vi "Read TSP Net Remote Instrument Data.vi"(7 "Enable Data Check (T: Enable)":bool=TRUE, 8 "error in (no error)":errorcluster, 9 "Data Format (Nil)":string="Nil", 10 "Instrument ID":string, 11 "VISA resource name":refnum<visa-resource-name>) -> (0 "error out":errorcluster, 2 "Remote Data":string, 3 "VISA resource name out":refnum<visa-resource-name>)   [LabVIEW 2017, in "Keithley 2600 Series.lvlib"]
doc: "Returns the data from the remote instrument.\n\n<b>Note:</b>\nThis VI only applies to the TSP-enabled instrument."
uses:
  <instrlib>/Keithley 2600 Series/Keithley 2600 Series.lvlib
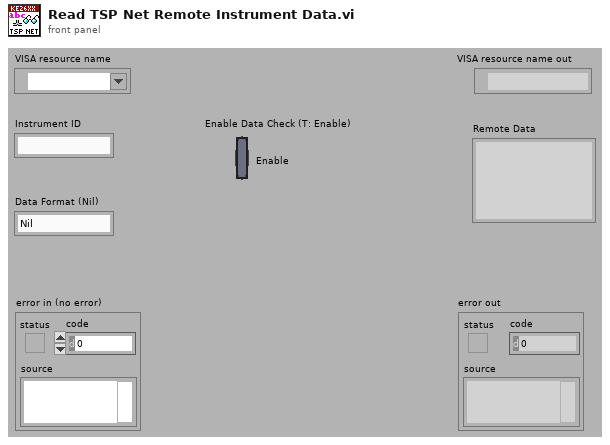
[diagram p1: front panel]
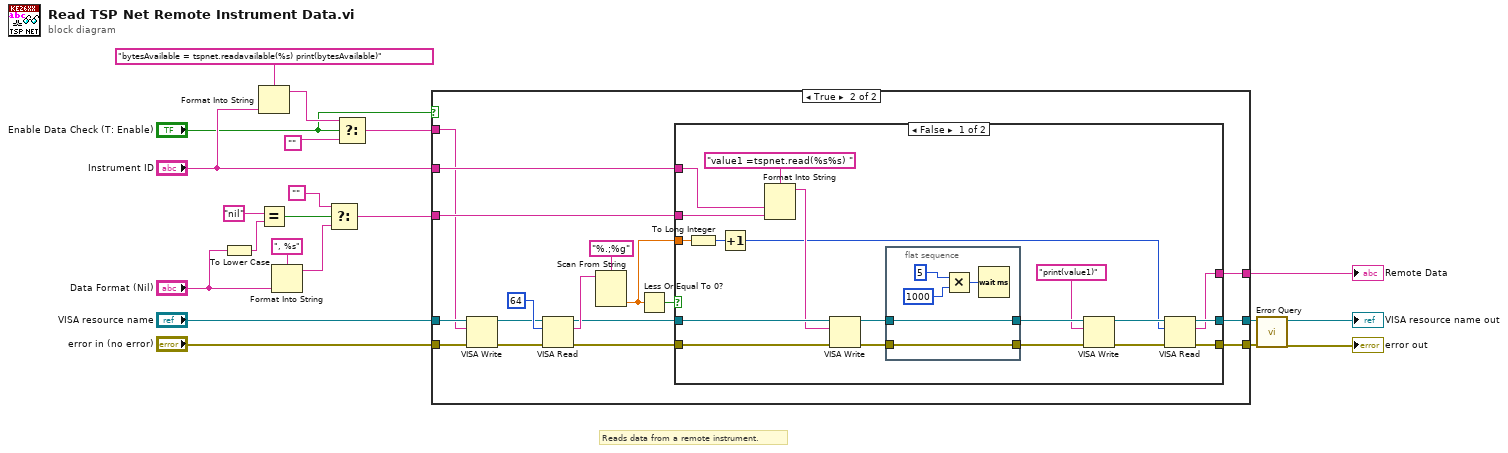
[diagram p0: block diagram]
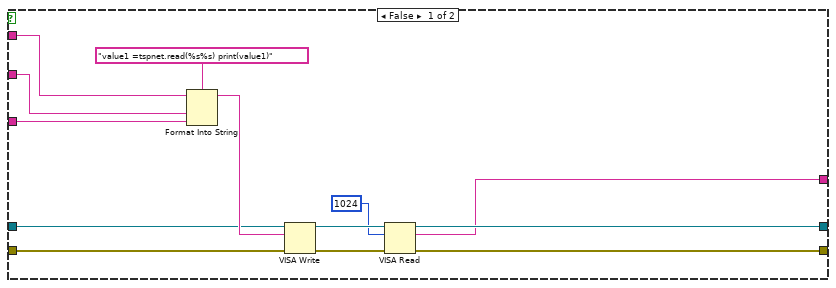
[diagram p2: hidden frame]
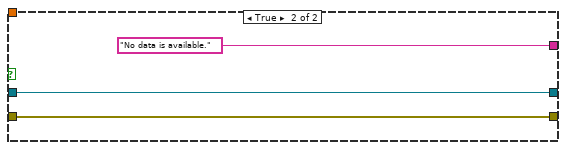
[diagram p3: hidden frame]
diagram:
  # "Reads data from a remote instrument."
  n1 = To Lower Case(string="Data Format (Nil)") -> (all lower case string=w2:string)
  n2 = Format Into String(format string="bytesAvailable = tspnet.readavailable(%s) print(bytesAvailable)", "Instrument ID") -> (resulting string=w18:string)  [unwired: 2 in, 1 out]
  n3 = Equal?(x="nil", y=w2) -> (x = y?=w14:bool)
  n4 = Format Into String(format string=", %s", "Data Format (Nil)") -> (resulting string=w11:string)  [unwired: 2 in, 1 out]
  n5 = Select(t="", s=w14, f=w11) -> (s? t:f=w10:string)
  n6 = Select(t=w18, s="Enable Data Check (T: Enable)", f="") -> (s? t:f=w5:string)
  n7 = case shown="True" "Enable Data Check (T: Enable)" {
    tunnel: "Instrument ID" -> [w23 w45]
    tunnel: w10 -> [w22 w44]
    tunnel: [w27 w43] -> w9
    tunnel: [w26 w42] -> w8
    tunnel: [w25 w41] -> w7
    tunnel: w5 -> [w24 w36]
    tunnel: "VISA resource name" -> [w29 w40]
    tunnel: "error in (no error)" -> [w28 w38]
    frame False {
      n8 = Format Into String(format string="value1 =tspnet.read(%s%s) print(value1)", initial string=w24, w23, w22) -> (resulting string=w30:string)  [unwired: 1 in, 1 out]
      n9 = VISA Write(VISA resource name=w29, write buffer=w30, error in (no error)=w28) -> (VISA resource name out=w33:refnum<visa-resource-name>, error out=w32:errorcluster)  [unwired: 1 out]
      n10 = VISA Read(VISA resource name=w33, byte count=u32 1024, error in (no error)=w32) -> (VISA resource name out=w27:refnum<visa-resource-name>, read buffer=w25:string, error out=w26:errorcluster)  [unwired: 1 out]
    }
    frame True {
      n11 = VISA Write(VISA resource name=w40, write buffer=w36, error in (no error)=w38) -> (VISA resource name out=w39:refnum<visa-resource-name>, error out=w37:errorcluster)  [unwired: 1 out]
      n12 = VISA Read(VISA resource name=w39, byte count=u32 64, error in (no error)=w37) -> (VISA resource name out=w47:refnum<visa-resource-name>, read buffer=w50:string, error out=w46:errorcluster)  [unwired: 1 out]
      n13 = Scan From String(format string="%.;%g", input string=w50) -> (output 1=w35:dbl)  [unwired: 3 in, 3 out]
      n14 = Less Or Equal To 0?(x=w35) -> (x <= 0?=w48:bool)
      n15 = case shown="False" w48 {
        tunnel: w47 -> [w67 w78]
        tunnel: w46 -> [w66 w77]
        tunnel: w45 -> [w69 _]
        tunnel: w44 -> [w68 _]
        tunnel: [w65 w78] -> w43
        tunnel: [w64 w77] -> w42
        tunnel: [w62 "No data is available." ("read buffer")] -> w41
        tunnel: w35 -> [w54 _]
        frame False {
          n16 = To Long Integer(number=w54) -> (32bit integer=w53:i32)
          n17 = Increment(x=w53) -> (x+1=w52:i32)
          n18 = Format Into String(format string="value1 =tspnet.read(%s%s) ", w69, w68) -> (resulting string=w63:string)  [unwired: 2 in, 1 out]
          n19 = VISA Write(VISA resource name=w67, write buffer=w63, error in (no error)=w66) -> (VISA resource name out=w61:refnum<visa-resource-name>, error out=w60:errorcluster)  [unwired: 1 out]
          n20 = flat-sequence {
            tunnel: w61 -> [w75]
            tunnel: w60 -> [w74]
            tunnel: [w75] -> w59
            tunnel: [w74] -> w57
            frame #0 {
              n21 = Multiply(x=5, y=1000) -> (x*y=w73:i32)
              n22 = Wait (ms)(milliseconds to wait=w73) -> ()  [unwired: 1 out]
            }
          }
          n23 = VISA Write(VISA resource name=w59, write buffer="print(value1)", error in (no error)=w57) -> (VISA resource name out=w58:refnum<visa-resource-name>, error out=w56:errorcluster)  [unwired: 1 out]
          n24 = VISA Read(VISA resource name=w58, byte count=w52, error in (no error)=w56) -> (VISA resource name out=w65:refnum<visa-resource-name>, read buffer=w62:string, error out=w64:errorcluster)  [unwired: 1 out]
        }
        frame True {
        }
      }
    }
  }
  "Remote Data" <- w7
  n25 = call <instrlib>:"Error Query.vi"("error in (no error)"=w8, "VISA resource name"=w9) -> ("error out"=→"error out":errorcluster, "VISA resource name out"=→"VISA resource name out":refnum<visa-resource-name>)  [unwired: 6 in, 2 out]
